vi "Build ToVSEngine Return Channels.vi"(8 "error in (no error)":errorcluster, 11 "Injector section ref in":T1 format="%.0x") -> (0 "error out":errorcluster, 2 "Results":T1[](array[typedef]) format="%.0x", 3 "Injector section ref out":T1 format="%.0x")   [LabVIEW 2019, in "Fuel Injector Analysis Addon System Explorer.lvlib"]
uses:
  Fuel Injector Analysis Addon System Explorer.lvlib
  <vilib>/NI VeriStand/Custom Device API/Custom Device Item Ref.ctl
  Addon Shared/Constants.vi
  <vilib>/NI VeriStand/Custom Device Tools/Custom Device Utility Library/NI VeriStand - Search for Item by GUID.vi
  <vilib>/NI VeriStand/Custom Device Tools/Custom Device Utility Library/NI VeriStand - Search for All Items by GUID.vi
  <vilib>/NI VeriStand/Custom Device Tools/Custom Device Utility Library/Custom Device Utility Library.lvlib
  Addon Shared/Fuel Injector Analysis Addon Shared.lvlib
  <vilib>/NI VeriStand/Custom Device API/Custom Device API.lvlib
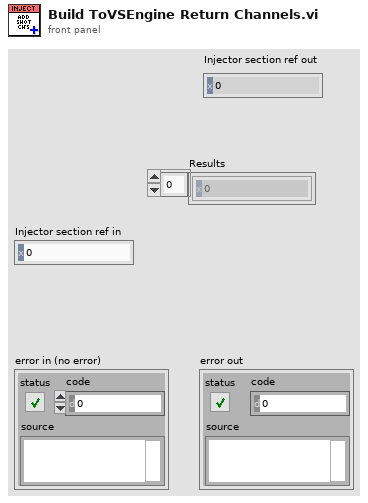
[diagram p1: front panel]
types:
  T1 = typedef "Custom Device API.lvlib/Custom Device Item Ref.ctl" = u64
  T2 = typedef "Custom Device API.lvlib/Custom Device Item Info.ctl" = cluster{"Name":string, "Is Channel":bool, "GUID":string, "Is Waveform":bool}
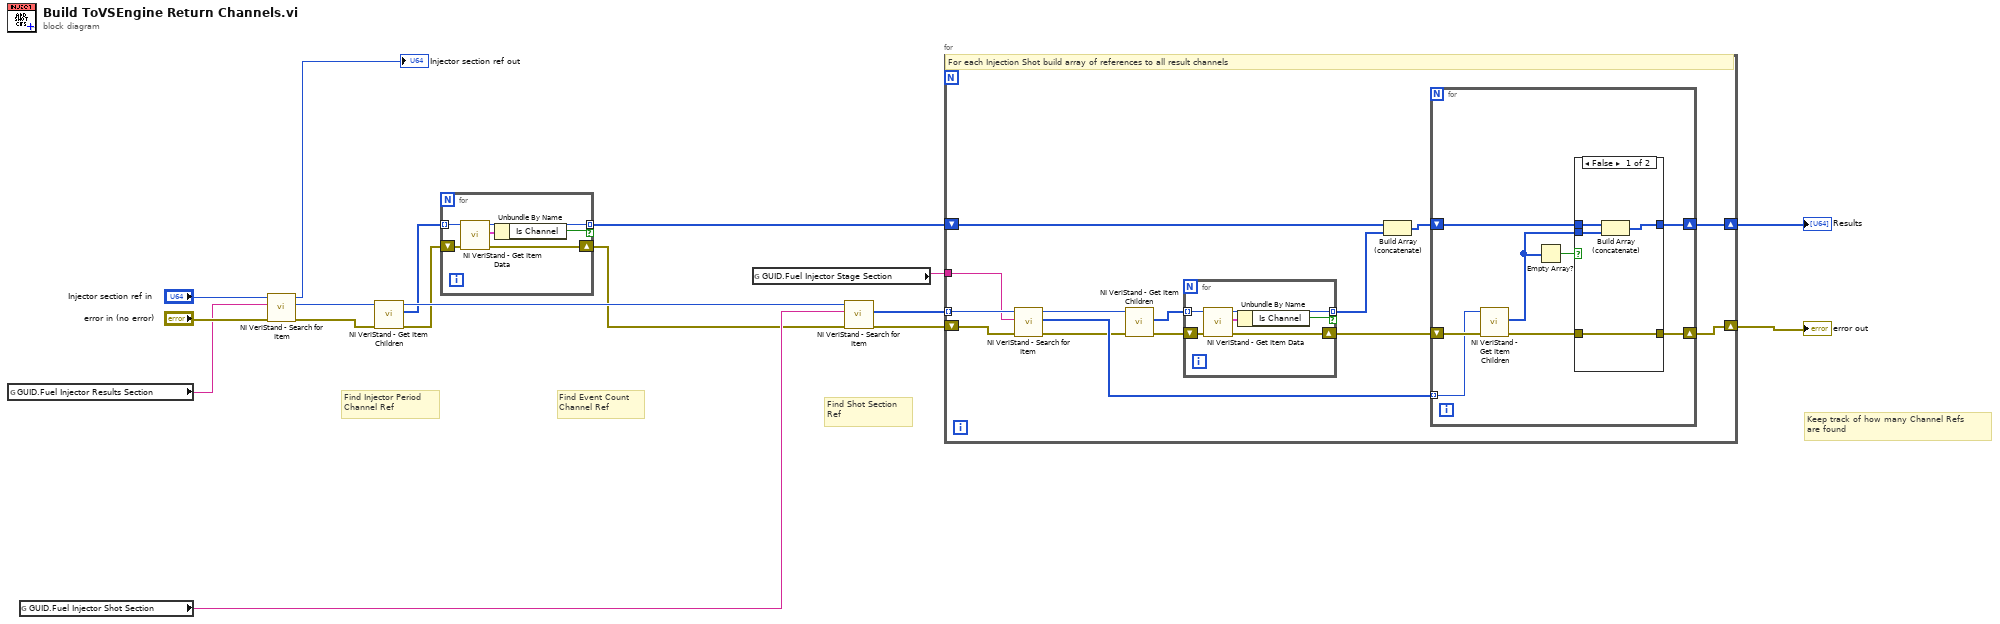
[diagram p0: block diagram]
diagram:
  # "Keep track of how many Channel Refs\nare found"
  # "Find Shot Section\nRef"
  # "Find Event Count\nChannel Ref"
  # "Find Injector Period\nChannel Ref"
  n1 = global read "Constants.vi" "GUID.Fuel Injector Results Section"() -> (w11:string)
  n2 = global read "Constants.vi" "GUID.Fuel Injector Shot Section"() -> (w15:string)
  n3 = call-poly <vilib>:"NI VeriStand - Search for Item.vi"("error in"="error in (no error)", "Item GUID"=w11, "Section Ref in"="Injector section ref in") -> ("error out"=w12:errorcluster, "Item Ref"=w10:T1, "Section Ref out"=→"Injector section ref out":T1)  [unwired: 5 in, 1 out]
  n4 = call <vilib>:"NI VeriStand - Get Item Children.vi"("error in (no error)"=w12, "Item Ref in"=w10) -> ("error out"=w2:errorcluster, "Child Refs"=w4:T1[], "Item Ref out"=w5:T1)  [unwired: 6 in, 1 out]
  n5 = for {
    tunnel: w4 -> [w23] mode=indexing
    tunnel: [w21] -> w3 mode=indexing if=w20
    shift-right: [w18] -> w1
    shift-left: w2 -> [w19]
    n6 = call <vilib>:"NI VeriStand - Get Item Data.vi"("error in (no error)"=w19, "Item Ref in"=w23) -> ("error out"=w18:errorcluster, "Item Info"=w22:T2, "Item Ref out"=w21:T1)  [unwired: 6 in, 1 out]
    n7 = Unbundle By Name(w22) -> ("Is Channel"=w20:bool)
  }
  n8 = global read "Constants.vi" "GUID.Fuel Injector Stage Section"() -> (w6:string)
  n9 = call-poly <vilib>:"NI VeriStand - Search for Item.vi"("error in"=w1, "Item GUID"=w15, "Section Ref in"=w5) -> ("error out"=w17:errorcluster, "Item Refs"=w16:T1[])  [unwired: 5 in, 2 out]
  n10 = for {
    tunnel: w16 -> [w37] mode=indexing
    shift-right: [w30] -> w14
    shift-left: w17 -> [w36]
    shift-right: [w34] -> w9
    shift-left: w3 -> [w35]
    tunnel: w6 -> [w33]
    # "For each Injection Shot build array of references to all result channels"
    n11 = call-poly <vilib>:"NI VeriStand - Search for Item.vi"("error in"=w36, "Item GUID"=w33, "Section Ref in"=w37) -> ("error out"=w27:errorcluster, "Item Refs"=w31:T1[], "Section Ref out"=w26:T1)  [unwired: 5 in, 1 out]
    n12 = call <vilib>:"NI VeriStand - Get Item Children.vi"("error in (no error)"=w27, "Item Ref in"=w26) -> ("error out"=w28:errorcluster, "Child Refs"=w29:T1[])  [unwired: 6 in, 2 out]
    n13 = for {
      tunnel: w29 -> [w43] mode=indexing
      tunnel: [w41] -> w25 mode=indexing if=w40
      shift-right: [w38] -> w24
      shift-left: w28 -> [w39]
      n14 = call <vilib>:"NI VeriStand - Get Item Data.vi"("error in (no error)"=w39, "Item Ref in"=w43) -> ("error out"=w38:errorcluster, "Item Info"=w42:T2, "Item Ref out"=w41:T1)  [unwired: 6 in, 1 out]
      n15 = Unbundle By Name(w42) -> ("Is Channel"=w40:bool)
    }
    n16 = Build Array (concatenate)(w35, w25) -> (w32:T1[])
    n17 = for {
      shift-right: [w49] -> w34
      shift-left: w32 -> [w51]
      tunnel: w31 -> [w47] mode=indexing
      shift-right: [w50] -> w30
      shift-left: w24 -> [w48]
      n18 = call <vilib>:"NI VeriStand - Get Item Children.vi"("error in (no error)"=w48, "Item Ref in"=w47) -> ("error out"=w46:errorcluster, "Child Refs"=w45:T1[])  [unwired: 6 in, 2 out]
      n19 = Empty Array?(array=w45) -> (empty?=w44:bool)
      n20 = case shown="False" w44 {
        tunnel: w51 -> [w55 w57]
        tunnel: w46 -> [w52 w56]
        tunnel: [w52 w56] -> w50
        tunnel: [w54 w57] -> w49
        tunnel: w45 -> [w53 _]
        frame False {
          n21 = Build Array (concatenate)(w55, w53) -> (w54:T1[])
        }
        frame True {
        }
      }
    }
  }
  "error out" <- w14
  "Results" <- w9
